vi "Send Configure Triggered Current Limit [TRG].vi"(7 "Message Priority (Normal)":T1=enum."Normal", 8 "error in (no error)":errorcluster, 9 "triggered limit (0.0 Amps)":dbl[unit] format="%^.2e", 10 "channel name (\"CHANNEL1\")":string="CHANNEL1", 11 "Message Enqueuer":refnum<class "Message Enqueuer.lvclass">) -> (0 "error out":errorcluster, 3 "Message Enqueuer out":refnum<class "Message Enqueuer.lvclass">)   [LabVIEW 2016, in "CS++DCPwr.lvlib" / "Configure Triggered Current Limit [TRG] Msg.lvclass"]
doc: "Sends the <B>CS++DCPwr.lvlib:Configure Triggered Current Limit [TRG] Msg.lvclass</B> message.\n\n<B>CS++DCPwr.lvlib:CS++DCPwr.lvclass:Configure Triggered Current Limit [TRG].vi</B> Description:\n\nThis VI configures the current limit the power supply uses after it receives a trigger.\n\nNotes:\n\n(1) This VI is part of the IviDCPwrTrigger [TRG] extension group."
uses:
  Configure Triggered Current Limit [TRG] Msg.lvclass
  <vilib>/ActorFramework/Message Enqueuer/Message Enqueuer.lvclass
  <vilib>/ActorFramework/Message Enqueuer/Message Priority.ctl
  C:/Program Files (x86)/National Instruments/LabVIEW 2016/vi.lib/ActorFramework/Message/Message.lvclass
  Configure Triggered Current Limit [TRG] Msg.lvclass/Configure Triggered Current Limit [TRG] Msg.ctl
  <vilib>/ActorFramework/Message Enqueuer/Message Enqueuer.lvclass/Message Enqueuer.ctl
  <vilib>/ActorFramework/Message Priority Queue/Priority Enqueue.vi
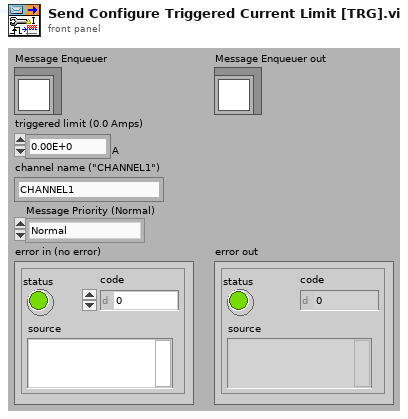
[diagram p1: front panel]
types:
  T1 = typedef "Actor Framework.lvlib/Message Enqueuer.lvclass/Message Priority.ctl" = enum16{"Low", "Normal", "High"}
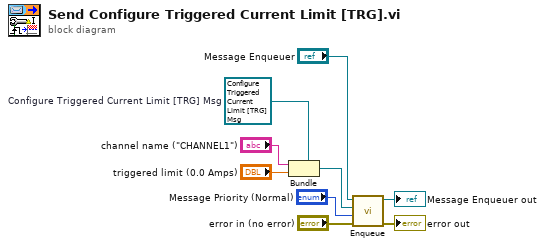
[diagram p0: block diagram]
diagram:
  w3 = refnum<class "Configure Triggered Current Limit [TRG] Msg.lvclass"> refnum  # Configure Triggered Current Limit [TRG] Msg
  n1 = Bundle(cluster=w3, "channel name (\"CHANNEL1\")", "triggered limit (0.0 Amps)") -> (w6:refnum<class "Configure Triggered Current Limit [TRG] Msg.lvclass">)
  n2 = call <vilib>:"Enqueue.vi"("error in (no error)"="error in (no error)", "Message Priority (Normal)"="Message Priority (Normal)", "Message"=w6, "Message Enqueuer in"="Message Enqueuer") -> ("error out"=→"error out":errorcluster, "Message Enqueuer out"=→"Message Enqueuer out":refnum<class "Message Enqueuer.lvclass">)  [unwired: 6 in]
